vi "svc_Complex Spectrum to Polar or Rectangular Components.vi"(2 "View":enum16{"Mag-Phase", "Real-Imaginary"}(ring), 4 "complex spectrum":cluster{"f0":dbl, "df":dbl, "spectrum":cdb[]} {"spectrum" format="%.2f"; "df" format="%.2f"; "f0" format="%.2f"}) -> (0 "phase or imaginary spectrum":cluster{"f0":dbl, "df":dbl, "spectrum":dbl[]} {"spectrum" format="%.2f"; "df" format="%.2f"; "f0" format="%.2f"}, 1 "magnitude or real spectrum":cluster{"f0":dbl, "df":dbl, "spectrum":dbl[]} {"spectrum" format="%.2f"; "df" format="%.2f"; "f0" format="%.2f"})   [LabVIEW 2017]
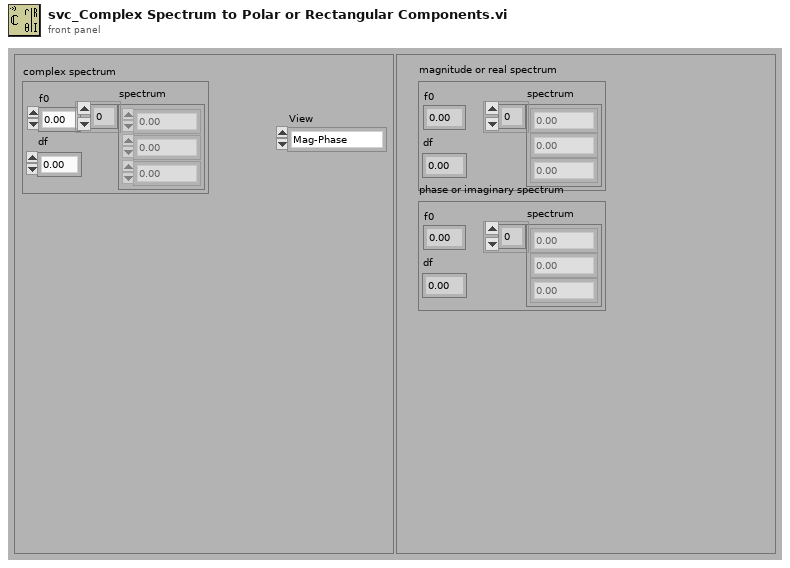
[diagram p1: front panel]
types:
  T1 = cluster{"f0":dbl, "df":dbl, "phase or imaginary part":dbl[]}
  T2 = cluster{"f0":dbl, "df":dbl, "magnitude or real part":dbl[]}
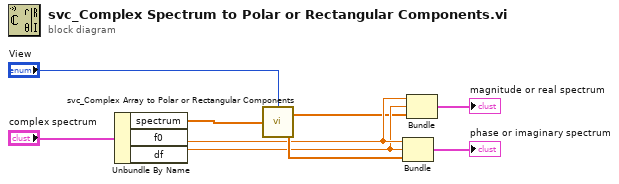
[diagram p0: block diagram]
diagram:
  n1 = Unbundle By Name("complex spectrum") -> ("spectrum"=w7:cdb[], "f0"=w4:dbl, "df"=w3:dbl)
  n2 = call <vilib>:"svc_Complex Array to Polar or Rectangular Components.vi"("View"="View", "complex array"=w7) -> ("phase or imaginary part"=w6:dbl[], "magnitude or real part"=w2:dbl[])  [unwired: 2 in]
  n3 = Bundle("f0"=w4, "df"=w3, "phase or imaginary part"=w6) -> (→"phase or imaginary spectrum":T1)  [unwired: 1 in]
  n4 = Bundle("f0"=w4, "df"=w3, "magnitude or real part"=w2) -> (→"magnitude or real spectrum":T2)  [unwired: 1 in]
